vi "003 ConvertidorGraus.vi"() -> ()   [LabVIEW 2019]
panel:
  out "Thermometer":dbl(slide) scale=-20.0..125.0
  out "Graus Fº":dbl
  in  "Graus Cº":dbl min=-273.0 max=273.0 step=1.0
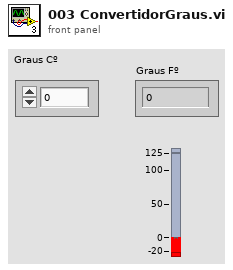
[diagram p1: front panel]
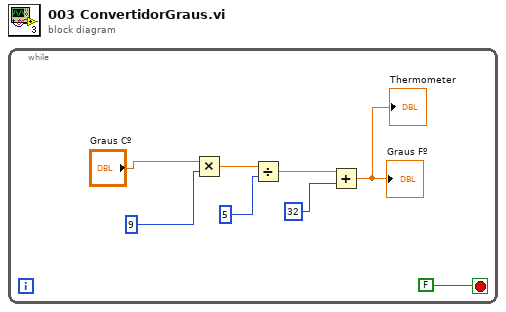
[diagram p0: block diagram]
diagram:
  n1 = while {
    stop <- FALSE stop-if-true
    n2 = Multiply(x="Graus Cº", y=9) -> (x*y=w6:dbl)
    n3 = Divide(x=w6, y=5) -> (x/y=w4:dbl)
    n4 = Add(x=w4, y=32) -> (x+y=→"Graus Fº" →"Thermometer":dbl)
  }
